vi "Validate Configuration (Plugin).vi"(8 "error in (no error)":errorcluster, 11 "plugin configuration in":T1={"name"="", "components"=[], "cycle timing"={"priority"=100, "decimation"=1, "offset"=0}, "threads"=[], "Transfer Groups"=[], "settings"=[]} {"Transfer Groups"."Transfers"."channels"."string offset" format="%d bytes"}) -> (0 "error out":errorcluster, 3 "plugin configuration out":T1={"name"="", "components"=[], "cycle timing"={"priority"=100, "decimation"=1, "offset"=0}, "threads"=[], "Transfer Groups"=[], "settings"=[]} {"Transfer Groups"."Transfers"."channels"."string offset" format="%d bytes"})   [LabVIEW 2017, in "DSF Core.lvlib" / "Configuration Session.lvclass"]
uses:
  Configuration Session.lvclass
  Typedefs/DSF Engine Plugin Configuration.ctl
  Typedefs/DSF Timing Info.ctl
  Typedefs/DSF Engine Plugin Thread Configuration.ctl
  Typedefs/DSF Settings Info.ctl
  Typedefs/DSF Engine Transfer Group Configuration.ctl
  Typedefs/DSF Direction.ctl
  Typedefs/DSF Engine Transfer Configuration.ctl
  Typedefs/DSF Byte Order.ctl
  Typedefs/DSF Engine Channel Configuration.ctl
  Typedefs/DSF Data Type.ctl
  Typedefs/DSF Timeout Behavior.ctl
  DSF Core.lvlib
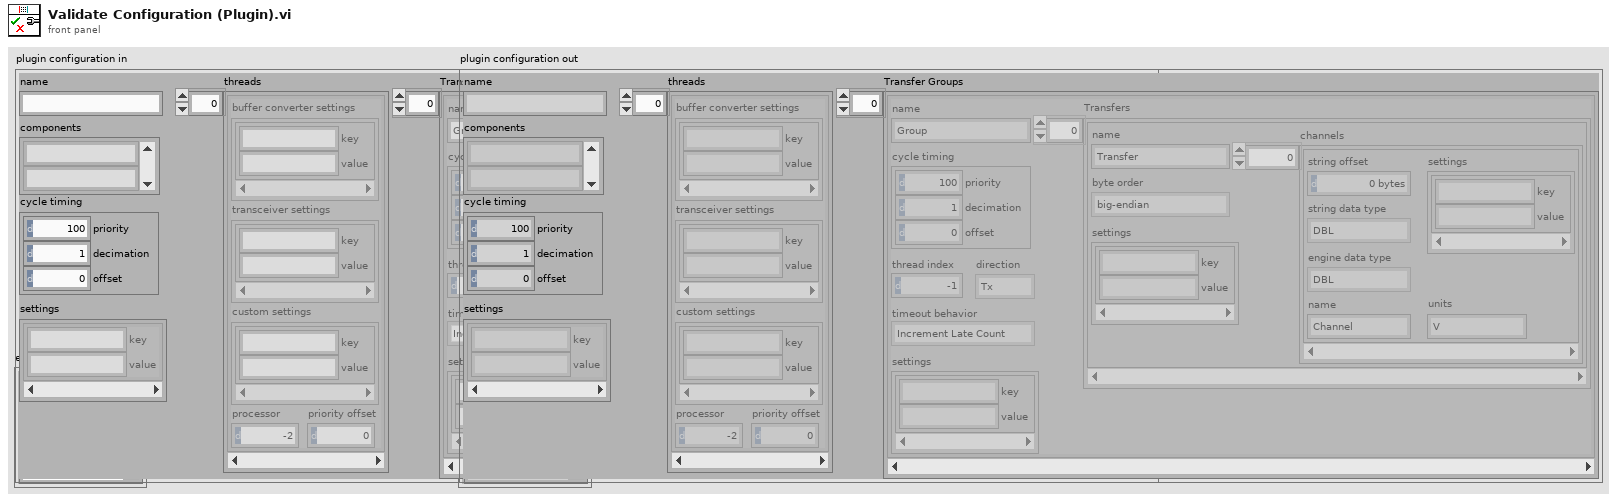
[diagram p1: front panel]
types:
  T1 = typedef "DSF Core.lvlib/DSF Engine Plugin Configuration.ctl" = cluster{"name":string, "components":string[], "cycle timing":T2, "threads":T3[], "Transfer Groups":T5[], "settings":T4}
  T2 = typedef "DSF Core.lvlib/DSF Timing Info.ctl" = cluster{"priority":u64, "decimation":u64, "offset":u64}
  T3 = typedef "DSF Core.lvlib/DSF Engine Plugin Thread Configuration.ctl" = cluster{"buffer converter settings":T4, "transceiver settings":T4, "custom settings":T4, "processor":i32, "priority offset":i16}
  T4 = typedef "DSF Core.lvlib/DSF Settings Info.ctl" = cluster{"key":string, "value":string}[]
  T5 = typedef "DSF Core.lvlib/DSF Engine Transfer Group Configuration.ctl" = cluster{"name":string, "direction":T6, "cycle timing":T2, "thread index":i32, "settings":T4, "Transfers":T7[], "timeout behavior":T11}
  T6 = typedef "DSF Core.lvlib/DSF Direction.ctl" = enum8{"Tx", "Rx"}
  T7 = typedef "DSF Core.lvlib/DSF Engine Transfer Configuration.ctl" = cluster{"name":string, "byte order":T8, "settings":T4, "channels":T9[]}
  T8 = typedef "DSF Core.lvlib/DSF Byte Order.ctl" = enum8{"big-endian", "little-endian"}
  T9 = typedef "DSF Core.lvlib/DSF Engine Channel Configuration.ctl" = cluster{"string offset":u64, "string data type":T10, "engine data type":T10, "name":string, "settings":T4, "units":string}
  T10 = typedef "DSF Core.lvlib/DSF Data Type.ctl" = enum8{"Bool", "SGL", "DBL", "I8", "I16", "I32", "I64", "U8", "U16", "U32", "U64"}
  T11 = typedef "DSF Core.lvlib/DSF Timeout Behavior.ctl" = enum8{"Increment Late Count", "Throw Error"}
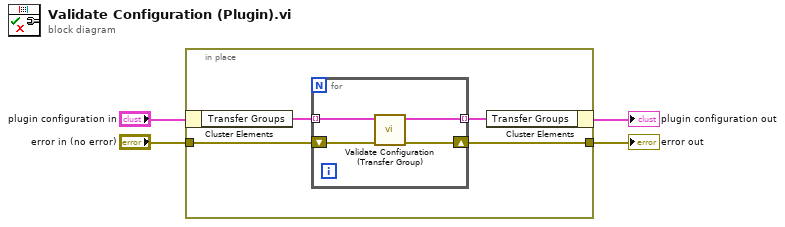
[diagram p0: block diagram]
diagram:
  n1 = in-place {
    in-place-border: "error in (no error)" -> [w6]
    in-place-border: [w5] -> w1
    n2 = in-place-cluster #1("plugin configuration in") -> ("Transfer Groups"=w8:T5[])
    n3 = for {
      tunnel: w8 -> [w12] mode=indexing
      tunnel: [w11] -> w7 mode=indexing
      shift-right: [w10] -> w5
      shift-left: w6 -> [w9]
      n4 = call "Validate Configuration (Transfer Group).vi"("error in (no error)"=w9, "transfer group configuration in"=w12) -> ("error out"=w10:errorcluster, "transfer group configuration out"=w11:T5)  [unwired: 8 in]
    }
    n5 = in-place-cluster #1("Transfer Groups"=w7) -> (→"plugin configuration out":T1)
  }
  "error out" <- w1
